vi "Read accounts.vi"(8 "error in":errorcluster, 10 "Users in":T1[](array[typedef]), 11 "filestatus":T2) -> (0 "error out":errorcluster, 3 "Users":T1[](array[typedef]))   [LabVIEW 2015]
doc: "Read/write user data from/to file."
uses:
  controls/user.ctl
  controls/filestatus.ctl
  <vilib>/Utility/file.llb/Write Delimited Spreadsheet (string).vi
  <vilib>/Utility/file.llb/Read Delimited Spreadsheet (string).vi
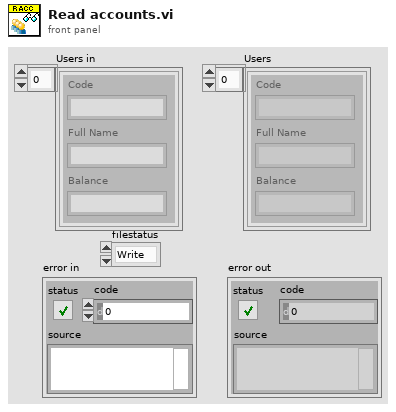
[diagram p1: front panel]
types:
  T1 = typedef "user.ctl" = cluster{"Code":string, "Full Name":string, "Balance":string}
  T2 = typedef "filestatus.ctl" = enum16{"Write", "Read"}
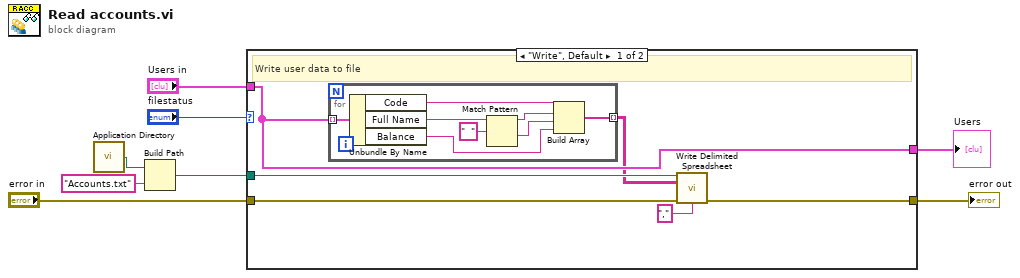
[diagram p0: block diagram]
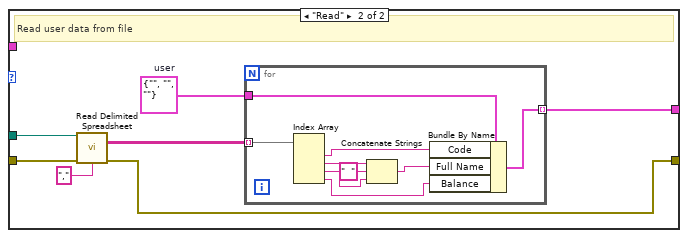
[diagram p2: hidden frame]
diagram:
  n1 = call <vilib>:"Application Directory.vi"() -> ("Application Directory"=w5:path)
  n2 = Build Path(base path=w5, name or relative path="Accounts.txt") -> (appended path=w6:path)
  n3 = case shown="\"Write\", Default" "filestatus" {
    tunnel: "error in" -> [w13 w29]
    tunnel: w6 -> [w12 w28]
    tunnel: [w10 w24] -> w3
    tunnel: "Users in" -> [w10 _]
    tunnel: [w11 w23] -> w1
    frame "Write", Default {
      # "Write user data to file"
      n4 = for {
        tunnel: w10 -> [w22] mode=indexing
        tunnel: [w15] -> w9 mode=indexing
        n5 = Unbundle By Name(w22) -> ("Code"=w19:string, "Full Name"=w21:string, "Balance"=w16:string)
        n6 = Match Pattern(string=w21, regular expression="  ") -> (before substring=w18:string, after substring=w17:string)  [unwired: 1 in, 2 out]
        n7 = Build Array(w19, w18, w17, w16) -> (w15:string[])
      }
      n8 = call-poly <vilib>:"Write Delimited Spreadsheet.vi"("file path (dialog if empty)"=w12, "2D data"=w9, "error in (no error)"=w13, "delimiter (\\t)"="," ("delimiter (\\t)")) -> ("error out"=w11:errorcluster)  [unwired: 10 in, 1 out]
    }
    frame "Read" {
      w25 = T1 {"Code"="", "Full Name"="", "Balance"=""}  # user
      # "Read user data from file"
      n9 = call-poly <vilib>:"Read Delimited Spreadsheet.vi"("file path (dialog if empty)"=w28, "error in (no error)"=w29, "delimiter (\\t)"="," ("delimiter (\\t)")) -> ("all rows"=w26:string[][], "error out"=w23:errorcluster)  [unwired: 7 in, 4 out]
      n10 = for {
        tunnel: w26 -> [w38] mode=indexing
        tunnel: w25 -> [w34]
        tunnel: [w30] -> w24 mode=indexing
        n11 = Index Array(array=w38) -> (element #1=w32:string, element #2=w37:string, element #3=w35:string, element #4=w33:string)  [unwired: 4 in]
        n12 = Concatenate Strings(w37, "  " ("string"), w35) -> (w31:string)
        n13 = Bundle By Name(cluster=w34, "Code"=w32, "Full Name"=w31, "Balance"=w33) -> (w30:T1)
      }
    }
  }
  "Users" <- w3
  "error out" <- w1
